vi "Read Actor FP Queue.vi"(11 "Template in":refnum<class "Template.lvclass">) -> (3 "Actor FP Queue":refnum<queue>)   [LabVIEW 2020, in "Template.lvlib" / "Template.lvclass"]
uses:
  Template.lvclass
  Template.lvclass/Template.ctl
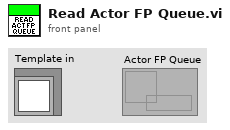
[diagram p1: front panel]
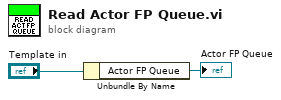
[diagram p0: block diagram]
diagram:
  n1 = Unbundle By Name("Template in") -> ("Actor FP Queue"=→"Actor FP Queue":refnum<queue>)
